vi "Update graph.vi"(4 "Load voltage deviation":dbl, 5 "Source Voltage":dbl, 6 "Load voltages":dbl, 7 "Buffer graph":bool, 9 "Efficiency":dbl, 10 "Load currents":dbl, 11 "UI in":T1={"Source Voltage[]"=[], "Old Load Current"=6.0, "EfficiencyGraph"=[], "LoadGraph(V/A)"=[], "LoadGraph(%)"=[], "Execution Time"=timestamp(0 s since 1904-01-01), "Debug file"=path ""}) -> (0 "LoadGraph(%)":T2(array[cluster]), 1 "LoadGraph(V/A)":T2(array[cluster]), 2 "EfficiencyGraph":T2(array[cluster]), 3 "UI out":T1={"Source Voltage[]"=[], "Old Load Current"=6.0, "EfficiencyGraph"=[], "LoadGraph(V/A)"=[], "LoadGraph(%)"=[], "Execution Time"=timestamp(0 s since 1904-01-01), "Debug file"=path ""})   [LabVIEW 2021, in "PMIC UI.lvlib"]
uses:
  PMIC UI.lvlib
  State Data.ctl
  <vilib>/Utility/file.llb/Write Delimited Spreadsheet (DBL).vi
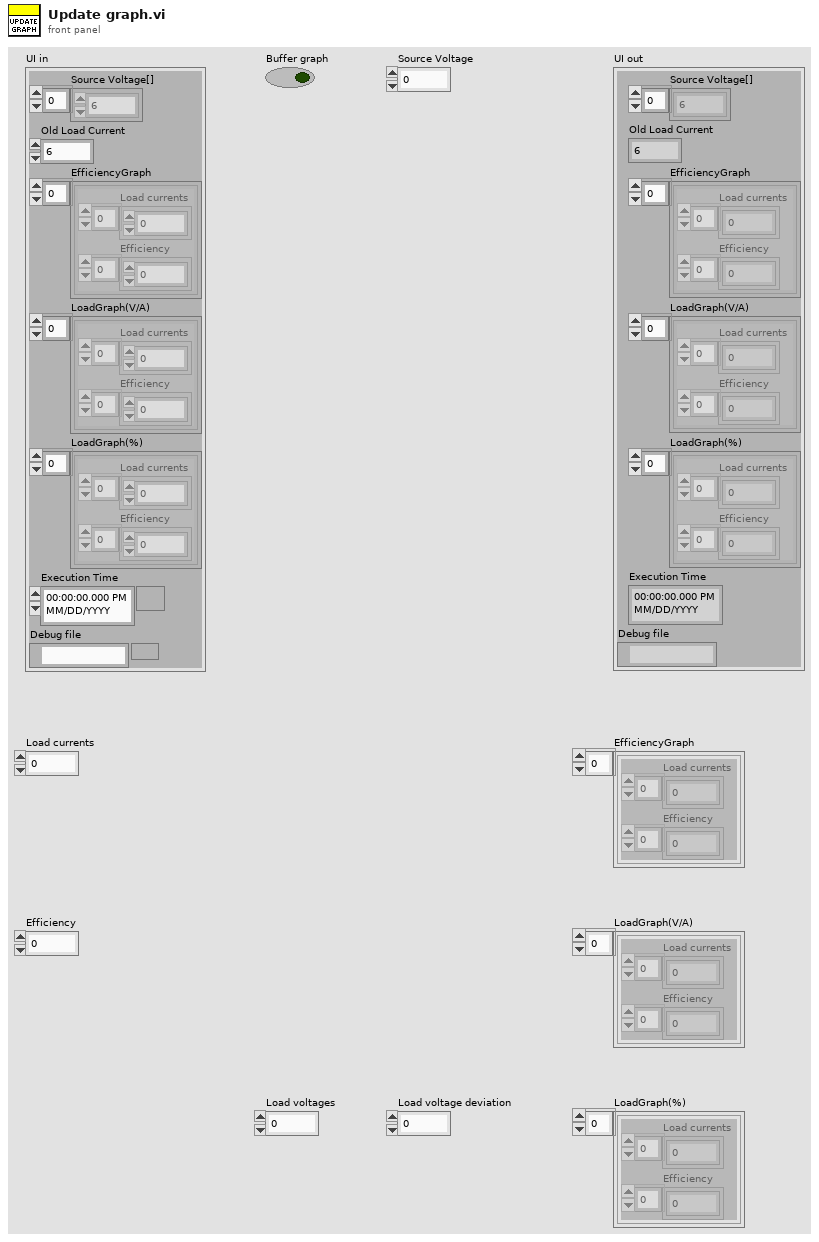
[diagram p1: front panel]
types:
  T1 = typedef "PMIC UI.lvlib/State Data.ctl" = cluster{"Source Voltage[]":dbl[], "Old Load Current":dbl, "EfficiencyGraph":cluster{"Load currents":dbl[], "Efficiency":dbl[]}[], "LoadGraph(V/A)":cluster{"Load currents":dbl[], "Efficiency":dbl[]}[], "LoadGraph(%)":cluster{"Load currents":dbl[], "Efficiency":dbl[]}[], "Execution Time":timestamp, "Debug file":path}
  T2 = cluster{"Load currents":dbl[], "Efficiency":dbl[]}[]
  T3 = cluster{"Load currents":dbl[], "Efficiency":dbl[]}
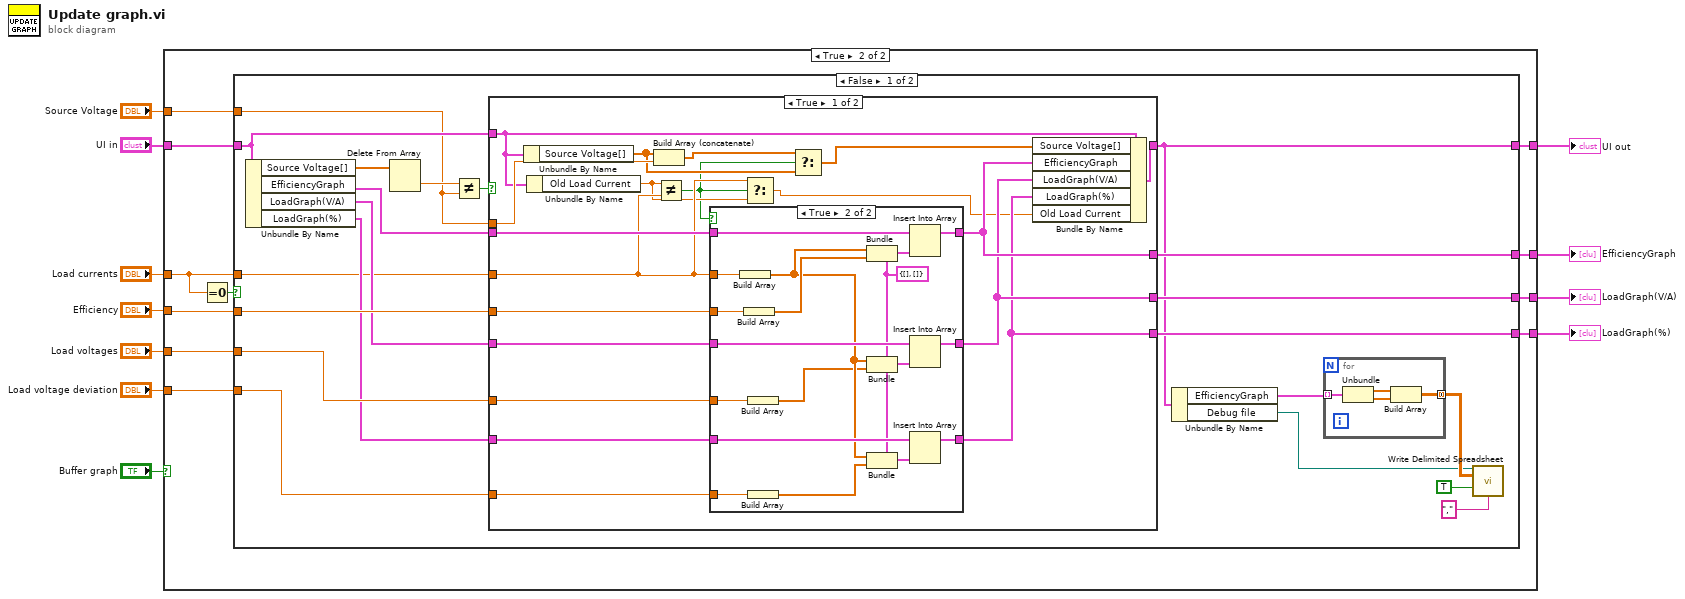
[diagram p0: block diagram]
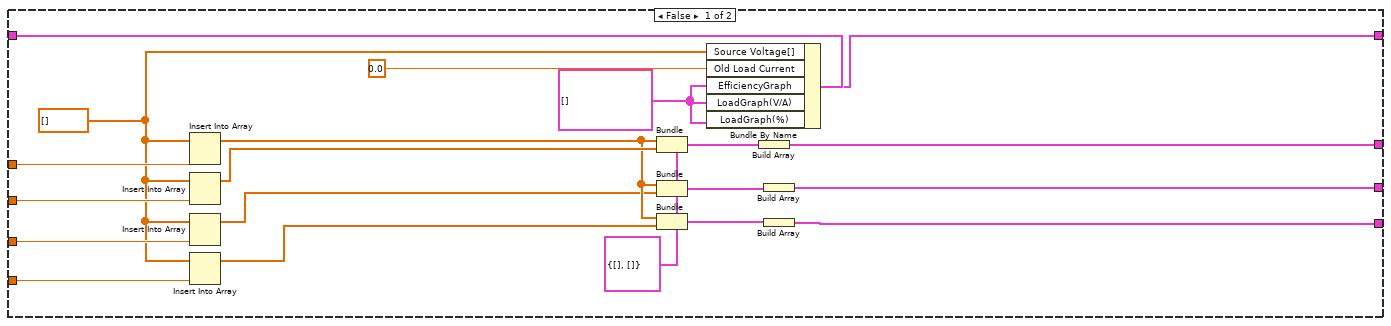
[diagram p2: hidden frame]
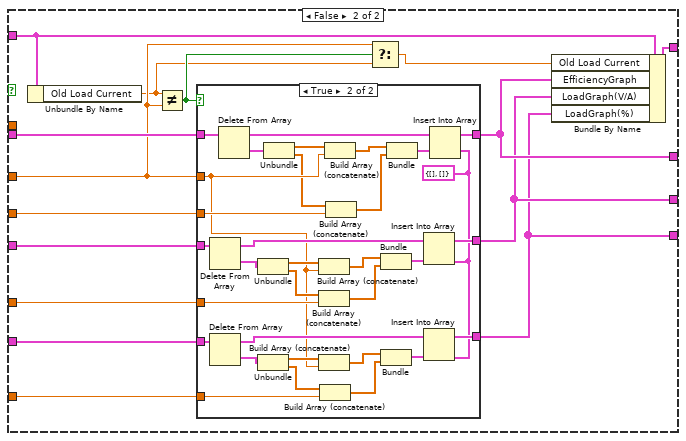
[diagram p4: hidden frame]
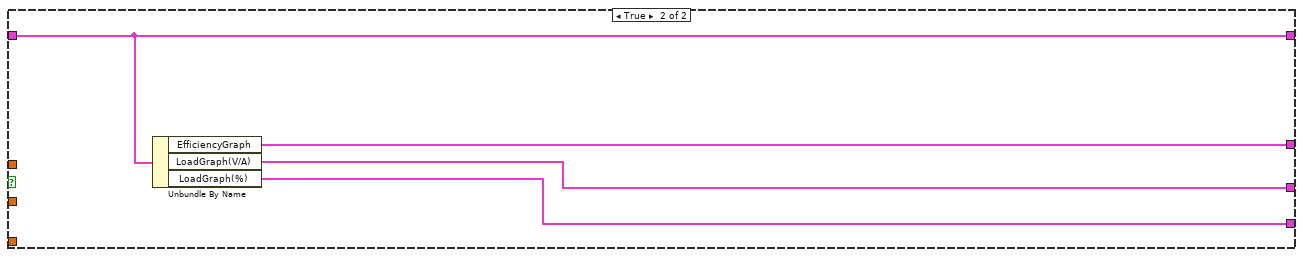
[diagram p6: hidden frame]
diagram:
  n1 = case shown="True" "Buffer graph" {
    tunnel: "UI in" -> [w27 w33]
    tunnel: "Load currents" -> [w31 w32]
    tunnel: "Efficiency" -> [w28 w42]
    tunnel: "Load voltages" -> [w23 w40]
    tunnel: "Load voltage deviation" -> [w22 w38]
    tunnel: [w29 w41] -> w10
    tunnel: [w25 w36] -> w7
    tunnel: [w15 w39] -> w8
    tunnel: [w14 w37] -> w9
    tunnel: "Source Voltage" -> [_ w35]
    frame False {
      w26 = T2 [] ("EfficiencyGraph")
      w17 = T3 {"Load currents"=[], "Efficiency"=[]} ("EfficiencyGraph")
      w13 = dbl[] [] ("Source Voltage")
      n2 = Insert Into Array(array=w13, new element=w31) -> (w21:dbl[])  [unwired: 1 in]
      n3 = Insert Into Array(array=w13, new element=w28) -> (w24:dbl[])  [unwired: 1 in]
      n4 = Insert Into Array(array=w13, new element=w23) -> (w20:dbl[])  [unwired: 1 in]
      n5 = Insert Into Array(array=w13, new element=w22) -> (w19:dbl[])  [unwired: 1 in]
      n6 = Bundle(cluster=w17, "Load currents"=w21, "Efficiency"=w24) -> (w30:T3)
      n7 = Bundle(cluster=w17, "Load currents"=w21, "Efficiency"=w20) -> (w18:T3)
      n8 = Bundle(cluster=w17, "Load currents"=w21, "Efficiency"=w19) -> (w16:T3)
      n9 = Bundle By Name(cluster=w27, "Source Voltage[]"=w13, "Old Load Current"=0.0 ("Old Load Voltage"), "EfficiencyGraph"=w26, "LoadGraph(V/A)"=w26, "LoadGraph(%)"=w26) -> (w25:T1)
      n10 = Build Array(w30) -> (w29:T2)
      n11 = Build Array(w18) -> (w15:T2)
      n12 = Build Array(w16) -> (w14:T2)
    }
    frame True {
      n13 = Equal To 0?(x=w32) -> (x = 0?=w34:bool)
      n14 = case shown="False" w34 {
        tunnel: w42 -> [w61 _]
        tunnel: [w60 w161] -> w41
        tunnel: w40 -> [w58 _]
        tunnel: [w57 w160] -> w39
        tunnel: w32 -> [w55 _]
        tunnel: w38 -> [w54 _]
        tunnel: [w53 w159] -> w37
        tunnel: [w45 w158] -> w36
        tunnel: w33 -> [w50 w158]
        tunnel: w35 -> [w49 _]
        frame False {
          n15 = Unbundle By Name(w50) -> ("Source Voltage[]"=w51:dbl[], "EfficiencyGraph"=w62:T2, "LoadGraph(V/A)"=w59:T2, "LoadGraph(%)"=w56:T2)
          n16 = Delete From Array(array=w51) -> (deleted portion=w63:dbl)  [unwired: 2 in, 1 out]
          n17 = Not Equal?(x=w63, y=w49) -> (x != y?=w52:bool)
          n18 = case shown="True" w52 {
            tunnel: w62 -> [w85 w113]
            tunnel: w61 -> [w86 w122]
            tunnel: [w79 w116] -> w60
            tunnel: w59 -> [w84 w121]
            tunnel: w58 -> [w83 w120]
            tunnel: [w78 w115] -> w57
            tunnel: w56 -> [w82 w119]
            tunnel: w55 -> [w74 w111]
            tunnel: w54 -> [w81 w118]
            tunnel: [w77 w114] -> w53
            tunnel: [w80 w117] -> w45
            tunnel: w50 -> [w75 w112]
            tunnel: w49 -> [w76 _]
            frame True {
              n19 = Unbundle By Name(w75) -> ("Source Voltage[]"=w71:dbl[])
              n20 = Unbundle By Name(w75) -> ("Old Load Current"=w73:dbl)
              n21 = Build Array (concatenate)(w71, w76) -> (w70:dbl[])
              n22 = Not Equal?(x=w73, y=w74) -> (x != y?=w69:bool)
              n23 = case shown="True" w69 {
                tunnel: w86 -> [_ w107]
                tunnel: w85 -> [w89 w105]
                tunnel: w84 -> [w88 w102]
                tunnel: w83 -> [_ w101]
                tunnel: w82 -> [w87 w100]
                tunnel: w81 -> [_ w98]
                tunnel: [w89 w94] -> w79
                tunnel: [w88 w93] -> w78
                tunnel: [w87 w92] -> w77
                tunnel: w74 -> [_ w90]
                frame False {
                }
                frame True {
                  w91 = cluster{dbl[], dbl[]} {[], []} ("cluster")
                  n24 = Build Array(w90) -> (w97:dbl[])
                  n25 = Build Array(w107) -> (w106:dbl[])
                  n26 = Build Array(w101) -> (w96:dbl[])
                  n27 = Build Array(w98) -> (w95:dbl[])
                  n28 = Bundle(cluster=w91, w97, w106) -> (w104:cluster{dbl[], dbl[]})
                  n29 = Bundle(cluster=w91, w97, w96) -> (w103:cluster{dbl[], dbl[]})
                  n30 = Bundle(cluster=w91, w97, w95) -> (w99:cluster{dbl[], dbl[]})
                  n31 = Insert Into Array(array=w105, new element=w104) -> (w94:T2)  [unwired: 1 in]
                  n32 = Insert Into Array(array=w102, new element=w103) -> (w93:T2)  [unwired: 1 in]
                  n33 = Insert Into Array(array=w100, new element=w99) -> (w92:T2)  [unwired: 1 in]
                }
              }
              n34 = Select(t=w74, s=w69, f=w73) -> (s? t:f=w72:dbl)
              n35 = Select(t=w70, s=w69, f=w71) -> (s? t:f=w68:dbl[])
              n36 = Bundle By Name(cluster=w75, "Source Voltage[]"=w68, "EfficiencyGraph"=w79, "LoadGraph(V/A)"=w78, "LoadGraph(%)"=w77, "Old Load Current"=w72) -> (w80:T1)
            }
            frame False {
              n37 = Unbundle By Name(w112) -> ("Old Load Current"=w108:dbl)
              n38 = Not Equal?(x=w108, y=w111) -> (x != y?=w109:bool)
              n39 = case shown="True" w109 {
                tunnel: w122 -> [_ w157]
                tunnel: w121 -> [w124 w149]
                tunnel: w120 -> [_ w148]
                tunnel: w119 -> [w123 w140]
                tunnel: w118 -> [_ w139]
                tunnel: [w125 w138] -> w116
                tunnel: [w124 w137] -> w115
                tunnel: [w123 w136] -> w114
                tunnel: w113 -> [w125 w135]
                tunnel: w111 -> [_ w134]
                frame False {
                }
                frame True {
                  w126 = cluster{dbl[], dbl[]} {[], []} ("cluster")
                  n40 = Delete From Array(array=w149) -> (deleted portion=w150:T3, array with subset deleted=w155:T2)  [unwired: 2 in]
                  n41 = Delete From Array(array=w140) -> (deleted portion=w147:T3, array with subset deleted=w142:T2)  [unwired: 2 in]
                  n42 = Delete From Array(array=w135) -> (deleted portion=w133:T3, array with subset deleted=w127:T2)  [unwired: 2 in]
                  n43 = Unbundle(w150) -> ("Load currents"=w151:dbl[], "Efficiency"=w152:dbl[])
                  n44 = Unbundle(w147) -> ("Load currents"=w146:dbl[], "Efficiency"=w145:dbl[])
                  n45 = Unbundle(w133) -> ("Load currents"=w132:dbl[], "Efficiency"=w131:dbl[])
                  n46 = Build Array (concatenate)(w151, w134) -> (w153:dbl[])
                  n47 = Build Array (concatenate)(w152, w148) -> (w154:dbl[])
                  n48 = Build Array (concatenate)(w146, w134) -> (w144:dbl[])
                  n49 = Build Array (concatenate)(w145, w139) -> (w143:dbl[])
                  n50 = Build Array (concatenate)(w132, w134) -> (w130:dbl[])
                  n51 = Build Array (concatenate)(w131, w157) -> (w129:dbl[])
                  n52 = Bundle(cluster=w126, w153, w154) -> (w156:cluster{dbl[], dbl[]})
                  n53 = Bundle(cluster=w126, w144, w143) -> (w141:cluster{dbl[], dbl[]})
                  n54 = Bundle(cluster=w126, w130, w129) -> (w128:cluster{dbl[], dbl[]})
                  n55 = Insert Into Array(array=w155, new element=w156) -> (w137:T2)  [unwired: 1 in]
                  n56 = Insert Into Array(array=w142, new element=w141) -> (w136:T2)  [unwired: 1 in]
                  n57 = Insert Into Array(array=w127, new element=w128) -> (w138:T2)  [unwired: 1 in]
                }
              }
              n58 = Select(t=w111, s=w109, f=w108) -> (s? t:f=w110:dbl)
              n59 = Bundle By Name(cluster=w112, "Old Load Current"=w110, "EfficiencyGraph"=w116, "LoadGraph(V/A)"=w115, "LoadGraph(%)"=w114) -> (w117:T1)
            }
          }
          n60 = Unbundle By Name(w45) -> ("EfficiencyGraph"=w44:T2, "Debug file"=w43:path)
          n61 = for {
            tunnel: w44 -> [w67] mode=indexing
            tunnel: [w64] -> w47 mode=concatenating
            n62 = Unbundle(w67) -> ("Load currents"=w66:dbl[], "Efficiency"=w65:dbl[])
            n63 = Build Array(w66, w65) -> (w64:dbl[][])
          }
          n64 = call-poly <vilib>:"Write Delimited Spreadsheet.vi"("file path (dialog if empty)"=w43, "2D data"=w47, "append to file? (new file:F)"=TRUE, "delimiter (\\t)"="," ("delimiter (\\t)")) -> ()  [unwired: 10 in, 2 out]
        }
        frame True {
          n65 = Unbundle By Name(w158) -> ("EfficiencyGraph"=w161:T2, "LoadGraph(V/A)"=w160:T2, "LoadGraph(%)"=w159:T2)
        }
      }
    }
  }
  "EfficiencyGraph" <- w10
  "LoadGraph(%)" <- w9
  "LoadGraph(V/A)" <- w8
  "UI out" <- w7
